vi "CloseCtlLookup.vi"(8 "error in (no error)":errorcluster, 11 "CtlLookup In":T1) -> (0 "error out":errorcluster)   [LabVIEW 2020, in "CtlReferences_API.lvlib"]
doc: "Close CtlLook up and clean-up"
uses:
  CtlReferences_API.lvlib
  CtlReferences/TypeDefs/CtlLookup.ctl
  CtlReferences/CtlReferences.lvclass
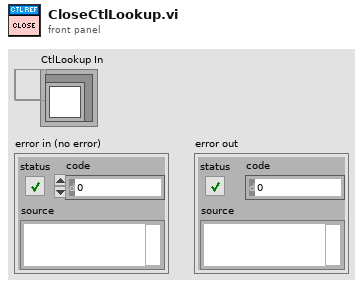
[diagram p1: front panel]
types:
  T1 = typedef "CtlReferences.lvlib/CtlReferences.lvclass/CtlLookup.ctl" = refnum<data-value>
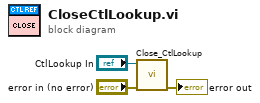
[diagram p0: block diagram]
diagram:
  n1 = call "Close_CtlLookup.vi"("error in (no error)"="error in (no error)", "CtlLookup In"="CtlLookup In") -> ("error out"=→"error out":errorcluster)  [unwired: 9 in]
